vi "Setup.vi"(8 "error in (no error)":errorcluster, 11 "FolloWin in":refnum<class "FolloWin.lvclass">) -> (0 "error out":errorcluster, 3 "FolloWin out":refnum<class "FolloWin.lvclass">)   [LabVIEW 2023, in "FolloWin.lvclass"]
doc: "Sets the FolloWin front panel properties and hides it (sets its transparency to 100)."
uses:
  FolloWin.lvclass
  <vilib>/Utility/miscctls.llb/LVPositionTypeDef.ctl
  FolloWin.lvclass/FolloWin.ctl
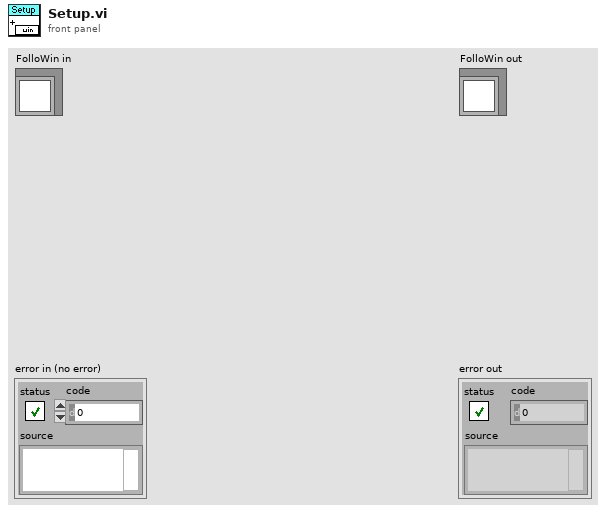
[diagram p1: front panel]
types:
  T1 = typedef "LVPositionTypeDef.ctl" = cluster{"Left":i32, "Top":i32}
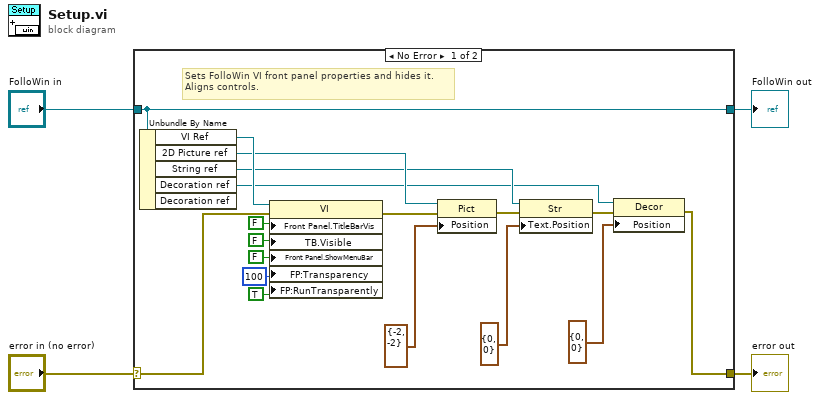
[diagram p0: block diagram]
diagram:
  n1 = case shown="No Error" "error in (no error)" {
    selector: "error in (no error)" -> [w15 w24]
    tunnel: [w6 w24] -> w3
    tunnel: [w17 w23] -> w1
    tunnel: "FolloWin in" -> [w17 w23]
    frame No Error {
      # "Sets FolloWin VI front panel properties and hides it.\nAligns controls."
      n2 = Unbundle By Name(w17) -> ("VI Ref"=w16:refnum<vi>, "2D Picture ref"=w14:refnum<vi>, "String ref"=w11:refnum<vi>, "Decoration ref"=w8:refnum<vi>)  [unwired: 1 out]
      n3 = property on="Property Node" class="VI"(reference=w16, error in=w15, "Front Panel.TitleBarVis"=FALSE ("Front Panel Window:Title Bar Visible"), "TB.Visible"=FALSE ("Tool Bar:Visible"), "Front Panel.ShowMenuBar"=FALSE ("Front Panel Window:Show Menu Bar"), "FP:Transparency"=u8 100 ("Front Panel Window:Transparency"), "FP:RunTransparently"=TRUE ("Front Panel Window:Run VI Transparently")) -> (error out=w13:errorcluster)  [unwired: 1 out]
      n4 = property class="Pict"(reference=w14, error in=w13, "Position"=T1 {"Left"=-2, "Top"=-2}) -> (error out=w12:errorcluster)  [unwired: 1 out]
      n5 = property class="Str"(reference=w11, error in=w12, "Text.Position"=T1 {"Left"=0, "Top"=0}) -> (error out=w9:errorcluster)  [unwired: 1 out]
      n6 = property class="Decor"(reference=w8, error in=w9, "Position"=T1 {"Left"=0, "Top"=0}) -> (error out=w6:errorcluster)  [unwired: 1 out]
    }
    frame Error {
    }
  }
  "error out" <- w3
  "FolloWin out" <- w1
